vi "Is in JKISM or CSM.vi"(8 "Error in":errorcluster caption="Error in (no error)", 11 "reference in":refnum<vi>) -> (0 "error out":errorcluster, 3 "is in JKISM or CSM?":bool)   [LabVIEW 2020, in "CSM-Helper.lvclass"]
uses:
  CSM-Helper.lvclass
  CSM-Helper.lvclass/CSM-Helper.ctl
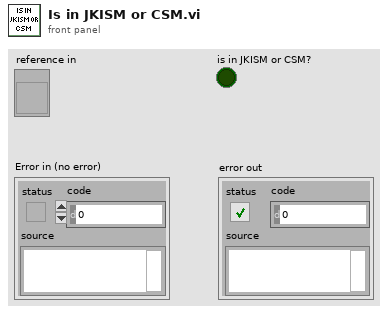
[diagram p1: front panel]
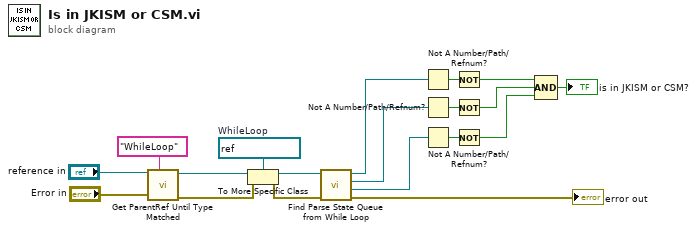
[diagram p0: block diagram]
diagram:
  w16 = refnum<vi> refnum  # WhileLoop
  n1 = call "Get ParentRef Until Type Matched.vi"("Class Name"="WhileLoop", "Error in"="Error in", "reference in"="reference in") -> ("Error out"=w14:errorcluster, "Target Ref"=w18:refnum<vi>)  [unwired: 5 in]
  n2 = To More Specific Class(target class=w16, reference=w18, error in=w14) -> (specific class reference=w17:refnum<vi>, error out=w15:errorcluster)
  n3 = call "Find Parse State Queue from While Loop.vi"("error in (no error)"=w15, "WhileLoop in"=w17) -> ("error out"=→"error out":errorcluster, "CaseStructure"=w6:refnum<vi>, "Parse State Queue"=w10:refnum<vi>, "WhileLoop out"=w5:refnum<vi>)  [unwired: 6 in]
  n4 = Not A Number/Path/Refnum?(number/path/refnum=w5) -> (NaN/Path/Refnum?=w8:bool)
  n5 = Not A Number/Path/Refnum?(number/path/refnum=w10) -> (NaN/Path/Refnum?=w9:bool)
  n6 = Not A Number/Path/Refnum?(number/path/refnum=w6) -> (NaN/Path/Refnum?=w7:bool)
  n7 = Not(x=w8) -> (.not. x?=w4:bool)
  n8 = Not(x=w9) -> (.not. x?=w3:bool)
  n9 = Not(x=w7) -> (.not. x?=w2:bool)
  n10 = Compound Arithmetic op=AND(w4, w3, w2) -> (→"is in JKISM or CSM?":bool)
